vi "All Columns Names.vi"() -> (0 "All column names":string[](array[string]))   [LabVIEW 2020, in "SignalConverson.lvlib"]
uses:
  SignalConverson.lvlib
  ScaledData.ctl
  Measrured TrapXYZ.ctl
  Data Before Angle Compensation.ctl
  Angle compensated data.ctl
  XYZ Signals.ctl
  Set TrapXYZ.ctl
  DAQChannelRawData.ctl
  Initialization/Physical Quantitites.ctl
  FlattenedData.ctl
  RingFlattenedData.ctl
panel:
  in  "RingFlattenedData defined by flattened data":u16(ring) items=["V_A' [V]", "V_D' [V]", "V_P'  [V]", "V_S' [V]", "V_L' [V]", "V_R' [V]", "V_sum' [V]", "V_x [V]", "V_y [V]", "V_px' [V]", "V_py' [V]", "V_pz' [V]", "dt [s]", "Vpx_AO [V]", "Vpy_AO [V]", "Vpz_AO [V]", "scan backlog", "LockInPhase", "TrapX [nm]", "TrapY [nm]", "TrapZ [nm]", "V_A [V]", "V_D [V]", "V_P [V]", "V_S [V]", "V_L [V]", "V_R [V]", "V_sum [V]", "V_x [V]", "V_y [V]", "P power [mW]", "S power [mW]", "angle compensated P power [W]", "angle compensated S power [W]", "angle compensated V_L", "angle compensated V_R", "angle compensated V_sum [V]", "angle compensated V_x [V]", "angle compensated V_y [V]", "Psi [rad]", "Laser power before objective[W]", "E_in", "E_out", "Delta E", "X signal", "Y signal", "Z signal", "TrapX (AO) [nm]", "TrapY (AO) [nm]", "TrapZ (AO) [nm]", "Fz [pN]", "Zext [nm]", "Tau [pNnm]", "Turn", "Fx [pN]", "Xext [nm]", "Fy [pN]", "Yext [nm]", "time [s]", "Delta Z signal", "Delta Z bead [nm]", "Z bead [nm]", "Delta TrapZ [nm]", "Delta Xsignal", "X bead [nm]", "Delta Ysignal", "Y bead [nm]", "Stop Condition"]
  in  "RingFlattenedData typeDef":T1 items=["V_A' [V]", "V_D' [V]", "V_P'  [V]", "V_S' [V]", "V_L' [V]", "V_R' [V]", "V_sum' [V]", "V_x [V]", "V_y [V]", "V_px' [V]", "V_py' [V]", "V_pz' [V]", "dt [s]", "Vpx_AO [V]", "Vpy_AO [V]", "Vpz_AO [V]", "scan backlog", "LockInPhase", "TrapX [nm]", "TrapY [nm]", "TrapZ [nm]", "V_A [V]", "V_D [V]", "V_P [V]", "V_S [V]", "V_L [V]", "V_R [V]", "V_sum [V]", "V_x [V]", "V_y [V]", "P power [mW]", "S power [mW]", "angle compensated P power [W]", "angle compensated S power [W]", "angle compensated V_L", "angle compensated V_R", "angle compensated V_sum [V]", "angle compensated V_x [V]", "angle compensated V_y [V]", "Psi [rad]", "Laser power before objective[W]", "E_in", "E_out", "Delta E", "X signal", "Y signal", "Z signal", "TrapX (AO) [nm]", "TrapY (AO) [nm]", "TrapZ (AO) [nm]", "Fz [pN]", "Zext [nm]", "Tau [pNnm]", "Turn", "Fx [pN]", "Xext [nm]", "Fy [pN]", "Yext [nm]", "time [s]", "Delta Z signal", "Delta Z bead [nm]", "Z bead [nm]", "Delta TrapZ [nm]", "Delta Xsignal", "X bead [nm]", "Delta Ysignal", "Y bead [nm]", "Stop Condition"]
  in  "RingFlattenedData":u16(ring) items=["V_A' [V]", "V_D' [V]", "V_P'  [V]", "V_S' [V]", "V_L' [V]", "V_R' [V]", "V_sum' [V]", "V_x [V]", "V_y [V]", "V_px' [V]", "V_py' [V]", "V_pz' [V]", "dt [s]", "Vpx_AO [V]", "Vpy_AO [V]", "Vpz_AO [V]", "scan backlog", "LockInPhase", "TrapX [nm]", "TrapY [nm]", "TrapZ [nm]", "V_A [V]", "V_D [V]", "V_P [V]", "V_S [V]", "V_L [V]", "V_R [V]", "V_sum [V]", "V_x [V]", "V_y [V]", "P power [mW]", "S power [mW]", "angle compensated P power [W]", "angle compensated S power [W]", "angle compensated V_L", "angle compensated V_R", "angle compensated V_sum [V]", "angle compensated V_x [V]", "angle compensated V_y [V]", "Psi [rad]", "Laser power before objective[W]", "E_in", "E_out", "Delta E", "X signal", "Y signal", "Z signal", "TrapX (AO) [nm]", "TrapY (AO) [nm]", "TrapZ (AO) [nm]", "Fz [pN]", "Zext [nm]", "Tau [pNnm]", "Turn", "Fx [pN]", "Xext [nm]", "Fy [pN]", "Yext [nm]", "time [s]", "Delta Z signal", "Delta Z bead [nm]", "Z bead [nm]", "Delta TrapZ [nm]", "Delta Xsignal", "X bead [nm]", "Delta Ysignal", "Y bead [nm]", "Stop Condition"]
  out "x = y?":bool[](array[boolean])
  out "All column names combined":string[](array[string])
  in  "Flattened data":T2
  out "size(s)":i32
  in  "Physical Quantities":T3
  out "c5":T4
  out "c4":T5
  out "c3":T6
  out "c2":T7
  out "c1":T8
  out "All column names from flattened data":string[](array[string])
  in  "ChannelNameArray":T9
  in  "All data after scaling":T10
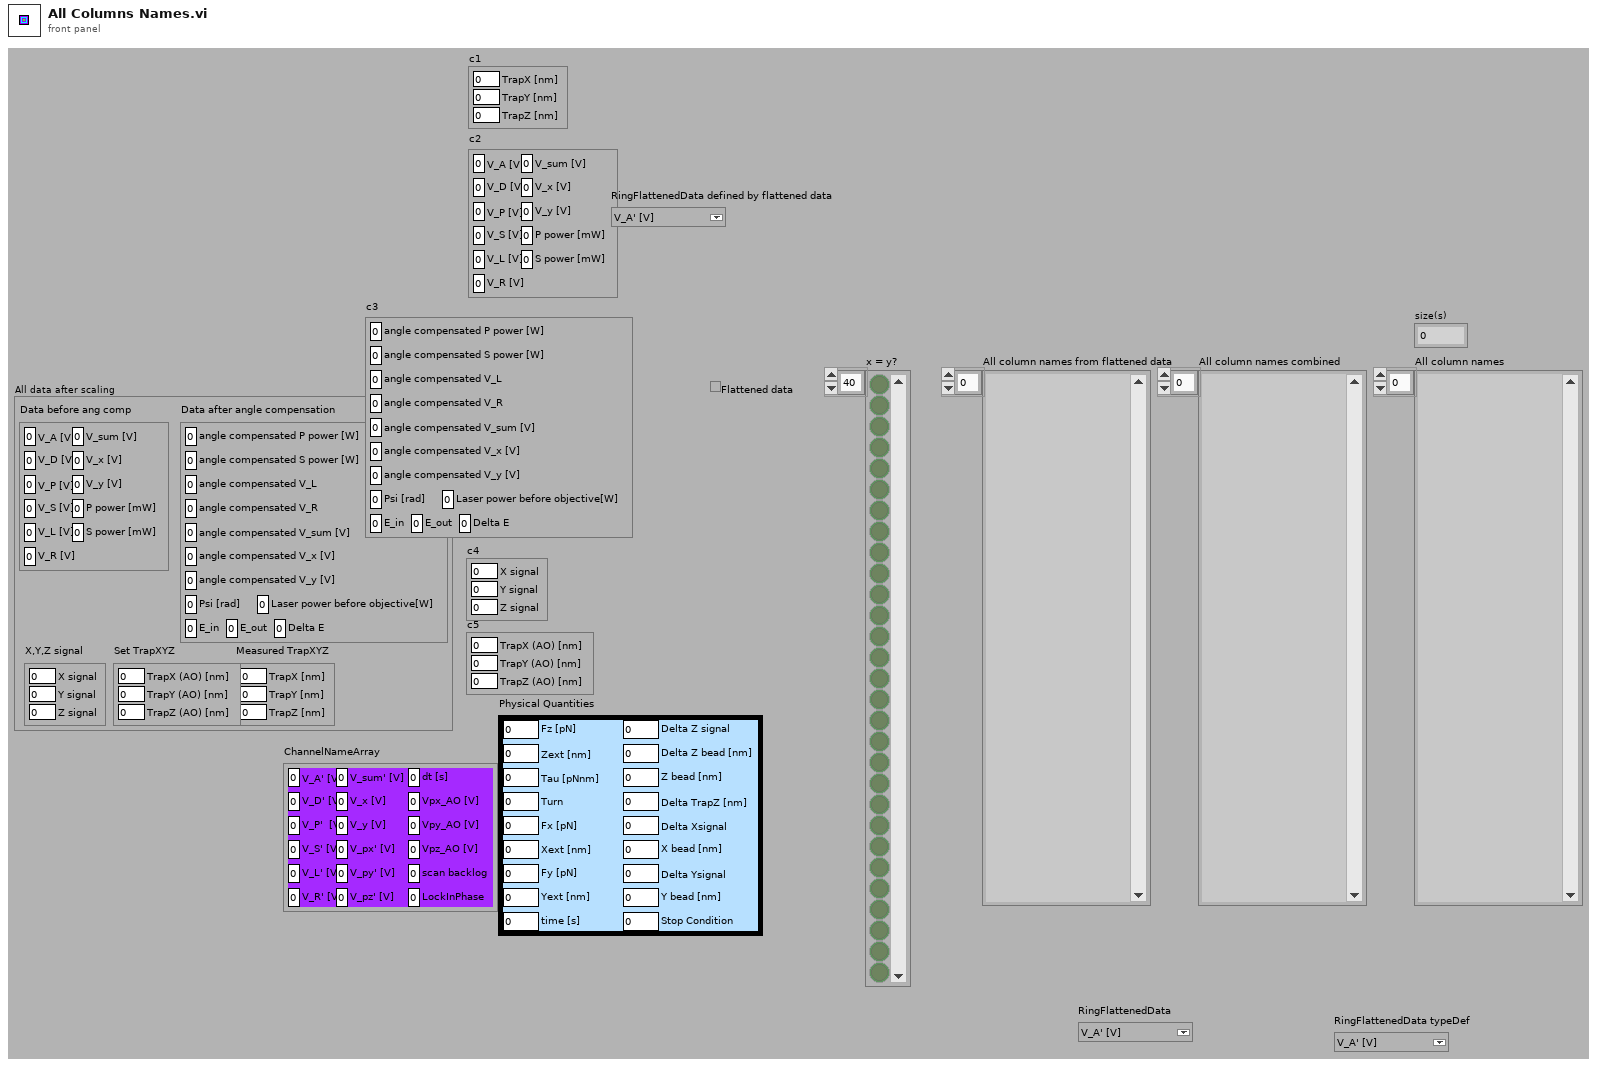
[diagram p1: front panel]
types:
  T1 = typedef "SignalConverson.lvlib/RingFlattenedData.ctl" = u16
  T2 = typedef "SignalConverson.lvlib/FlattenedData.ctl" = cluster{"V_A' [V]":dbl, "V_D' [V]":dbl, "V_P'  [V]":dbl, "V_S' [V]":dbl, "V_L' [V]":dbl, "V_R' [V]":dbl, "V_sum' [V]":dbl, "V_x [V]":dbl, "V_y [V]":dbl, "V_px' [V]":dbl, "V_py' [V]":dbl, "V_pz' [V]":dbl, "dt [s]":dbl, "Vpx_AO [V]":dbl, "Vpy_AO [V]":dbl, "Vpz_AO [V]":dbl, "scan backlog":dbl, "LockInPhase":dbl, "TrapX [nm]":dbl, "TrapY [nm]":dbl, "TrapZ [nm]":dbl, "V_A [V]":dbl, "V_D [V]":dbl, "V_P [V]":dbl, "V_S [V]":dbl, "V_L [V]":dbl, "V_R [V]":dbl, "V_sum [V]":dbl, "V_x [V]":dbl, "V_y [V]":dbl, "P power [mW]":dbl, "S power [mW]":dbl, "angle compensated P power [W]":dbl, "angle compensated S power [W]":dbl, "angle compensated V_L":dbl, "angle compensated V_R":dbl, "angle compensated V_sum [V]":dbl, "angle compensated V_x [V]":dbl, "angle compensated V_y [V]":dbl, "Psi [rad]":dbl, "Laser power before objective[W]":dbl, "E_in":dbl, "E_out":dbl, "Delta E":dbl, "X signal":dbl, "Y signal":dbl, "Z signal":dbl, "TrapX (AO) [nm]":dbl, "TrapY (AO) [nm]":dbl, "TrapZ (AO) [nm]":dbl, "Fz [pN]":dbl, "Zext [nm]":dbl, "Tau [pNnm]":dbl, "Turn":dbl, "Fx [pN]":dbl, "Xext [nm]":dbl, "Fy [pN]":dbl, "Yext [nm]":dbl, "time [s]":dbl, "Delta Z signal":dbl, "Delta Z bead [nm]":dbl, "Z bead [nm]":dbl, "Delta TrapZ [nm]":dbl, "Delta Xsignal":dbl, "X bead [nm]":dbl, "Delta Ysignal":dbl, "Y bead [nm]":dbl, "Stop Condition":dbl}
  T3 = typedef "SignalConverson.lvlib/Physical Quantitites.ctl" = cluster{"Fz [pN]":dbl, "Zext [nm]":dbl, "Tau [pNnm]":dbl, "Turn":dbl, "Fx [pN]":dbl, "Xext [nm]":dbl, "Fy [pN]":dbl, "Yext [nm]":dbl, "time [s]":dbl, "Delta Z signal":dbl, "Delta Z bead [nm]":dbl, "Z bead [nm]":dbl, "Delta TrapZ [nm]":dbl, "Delta Xsignal":dbl, "X bead [nm]":dbl, "Delta Ysignal":dbl, "Y bead [nm]":dbl, "Stop Condition":dbl}
  T4 = typedef "SignalConverson.lvlib/Set TrapXYZ.ctl" = cluster{"TrapX (AO) [nm]":dbl, "TrapY (AO) [nm]":dbl, "TrapZ (AO) [nm]":dbl}
  T5 = typedef "SignalConverson.lvlib/XYZ Signals.ctl" = cluster{"X signal":dbl, "Y signal":dbl, "Z signal":dbl}
  T6 = typedef "SignalConverson.lvlib/Angle compensated data.ctl" = cluster{"angle compensated P power [W]":dbl, "angle compensated S power [W]":dbl, "angle compensated V_L":dbl, "angle compensated V_R":dbl, "angle compensated V_sum [V]":dbl, "angle compensated V_x [V]":dbl, "angle compensated V_y [V]":dbl, "Psi [rad]":dbl, "Laser power before objective[W]":dbl, "E_in":dbl, "E_out":dbl, "Delta E":dbl}
  T7 = typedef "SignalConverson.lvlib/Data Before Angle Compensation.ctl" = cluster{"V_A [V]":dbl, "V_D [V]":dbl, "V_P [V]":dbl, "V_S [V]":dbl, "V_L [V]":dbl, "V_R [V]":dbl, "V_sum [V]":dbl, "V_x [V]":dbl, "V_y [V]":dbl, "P power [mW]":dbl, "S power [mW]":dbl}
  T8 = typedef "SignalConverson.lvlib/Measrured TrapXYZ.ctl" = cluster{"TrapX [nm]":dbl, "TrapY [nm]":dbl, "TrapZ [nm]":dbl}
  T9 = typedef "SignalConverson.lvlib/DAQChannelRawData.ctl" = cluster{"V_A' [V]":dbl, "V_D' [V]":dbl, "V_P'  [V]":dbl, "V_S' [V]":dbl, "V_L' [V]":dbl, "V_R' [V]":dbl, "V_sum' [V]":dbl, "V_x [V]":dbl, "V_y [V]":dbl, "V_px' [V]":dbl, "V_py' [V]":dbl, "V_pz' [V]":dbl, "dt [s]":dbl, "Vpx_AO [V]":dbl, "Vpy_AO [V]":dbl, "Vpz_AO [V]":dbl, "scan backlog":u32, "LockInPhase":dbl}
  T10 = typedef "SignalConverson.lvlib/ScaledData.ctl" = cluster{"Measured TrapXYZ":T8, "Data before ang comp":T7, "Data after angle compensation":T6, "X,Y,Z signal":T5, "Set TrapXYZ":T4}
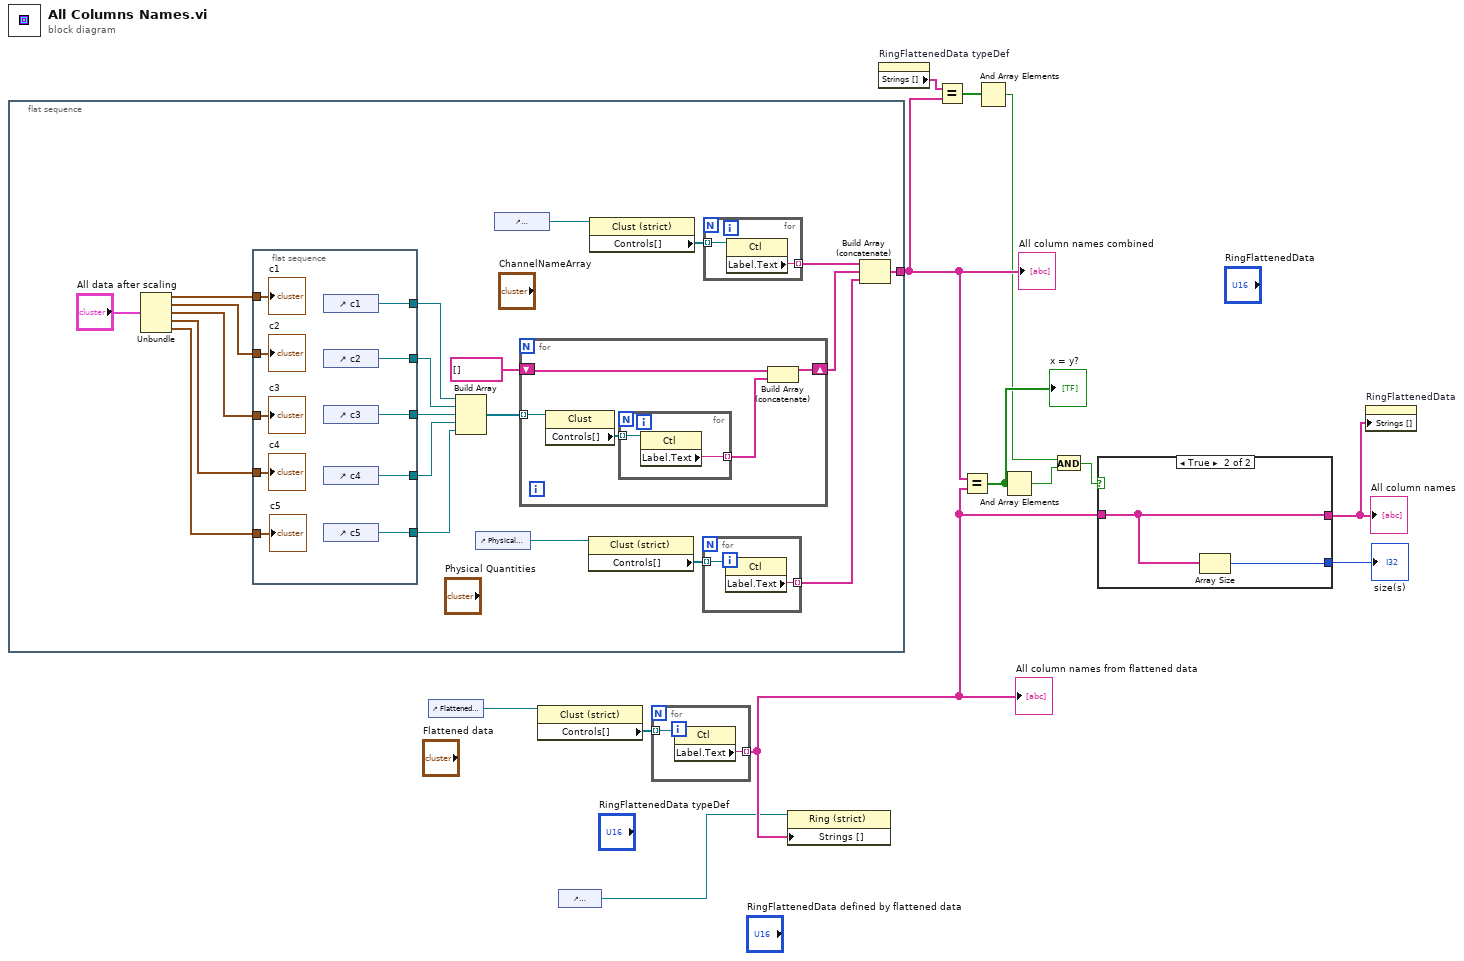
[diagram p0: block diagram]
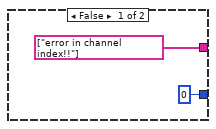
[diagram p2: hidden frame]
diagram:
  n1 = flat-sequence {
    tunnel: [w14] -> w7
    frame #0 {
      n2 = Unbundle("All data after scaling") -> ("Measured TrapXYZ"=w30:T8, "Data before ang comp"=w29:T7, "Data after angle compensation"=w28:T6, "X,Y,Z signal"=w27:T5, "Set TrapXYZ"=w26:T4)
      n3 = flat-sequence {
        tunnel: w30 -> [w46]
        tunnel: w29 -> [w45]
        tunnel: w28 -> [w44]
        tunnel: w27 -> [w43]
        tunnel: w26 -> [w42]
        tunnel: [w41] -> w25
        tunnel: [w40] -> w24
        tunnel: [w39] -> w23
        tunnel: [w38] -> w22
        tunnel: [w37] -> w21
        frame #0 {
          n4 = control-ref of="c1"() -> (w41:refnum<vi>)
          n5 = control-ref of="c2"() -> (w40:refnum<vi>)
          n6 = control-ref of="c3"() -> (w39:refnum<vi>)
          n7 = control-ref of="c4"() -> (w38:refnum<vi>)
          n8 = control-ref of="c5"() -> (w37:refnum<vi>)
          "c1" <- w46
          "c2" <- w45
          "c3" <- w44
          "c4" <- w43
          "c5" <- w42
        }
      }
      n9 = Build Array(w25, w24, w23, w22, w21) -> (w20:refnum<vi>[])
      n10 = control-ref of="Physical Quantities"() -> (w16:refnum<vi>)
      n11 = control-ref of="ChannelNameArray"() -> (w33:refnum<vi>)
      n12 = for {
        tunnel: w20 -> [w51] mode=indexing
        shift-right: [w48] -> w18
        shift-left: string[] [] -> [w47]
        n13 = property class="Clust"(reference=w51) -> ("Controls[]"=w50:refnum<vi>[])  [unwired: 1 in, 2 out]
        n14 = for {
          tunnel: w50 -> [w53] mode=indexing
          tunnel: [w52] -> w49 mode=indexing
          n15 = property class="Ctl"(reference=w53) -> ("Label.Text"=w52:string)  [unwired: 1 in, 2 out]
        }
        n16 = Build Array (concatenate)(w47, w49) -> (w48:string[])
      }
      n17 = property class="Clust (strict)"(reference=w16) -> ("Controls[]"=w17:refnum<vi>[])  [unwired: 1 in, 2 out]
      n18 = property class="Clust (strict)"(reference=w33) -> ("Controls[]"=w34:refnum<vi>[])  [unwired: 1 in, 2 out]
      n19 = for {
        tunnel: w17 -> [w36] mode=indexing
        tunnel: [w35] -> w15 mode=indexing
        n20 = property class="Ctl"(reference=w36) -> ("Label.Text"=w35:string)  [unwired: 1 in, 2 out]
      }
      n21 = for {
        tunnel: w34 -> [w55] mode=indexing
        tunnel: [w54] -> w32 mode=indexing
        n22 = property class="Ctl"(reference=w55) -> ("Label.Text"=w54:string)  [unwired: 1 in, 2 out]
      }
      n23 = Build Array (concatenate)(w32, w18, w15) -> (w14:string[])
    }
  }
  n24 = control-ref of="Flattened data"() -> (w12:refnum<vi>)
  n25 = property class="Clust (strict)"(reference=w12) -> ("Controls[]"=w13:refnum<vi>[])  [unwired: 1 in, 2 out]
  n26 = control-ref of="RingFlattenedData defined by flattened data"() -> (w1:refnum<vi>)
  n27 = for {
    tunnel: w13 -> [w57] mode=indexing
    tunnel: [w56] -> w2 mode=indexing
    n28 = property class="Ctl"(reference=w57) -> ("Label.Text"=w56:string)  [unwired: 1 in, 2 out]
  }
  "All column names from flattened data" <- w2
  n29 = property on="Property Node" class="Ring (strict)"(reference=w1, "Strings []"=w2) -> ()  [unwired: 1 in, 2 out]
  n30 = property on="RingFlattenedData typeDef" class="Ring (strict)"() -> ("Strings []"=w8:string[])  [unwired: 2 in, 2 out]
  n31 = Equal?(x=w8, y=w7) -> (x = y?=w6:bool[])
  n32 = Equal?(x=w7, y=w2) -> (x = y?=w11:bool[])
  "x = y?" <- w11
  n33 = And Array Elements(Boolean array=w6) -> (logical AND=w3:bool)
  n34 = And Array Elements(Boolean array=w11) -> (logical AND=w5:bool)
  n35 = And(x=w3, y=w5) -> (x .and. y?=w4:bool)
  n36 = case shown="True" w4 {
    tunnel: w2 -> [_ w61]
    tunnel: [string[] ["error in channel index!!"] w61] -> w9
    tunnel: [0 w60] -> w10
    frame False {
    }
    frame True {
      n37 = Array Size(array=w61) -> (size(s)=w60:i32)
    }
  }
  "size(s)" <- w10
  "All column names" <- w9
  n38 = property on="RingFlattenedData" class="Ring (strict)"("Strings []"=w9) -> ()  [unwired: 2 in, 2 out]
  "All column names combined" <- w7
